vi "counter_control.vi"(0 "Signal-high duration":u32=20, 1 "Signal-high lead-up":u32=10) -> ()   [LabVIEW 2010]
panel:
  out "Configuration Error messages":T1
  # "Output"
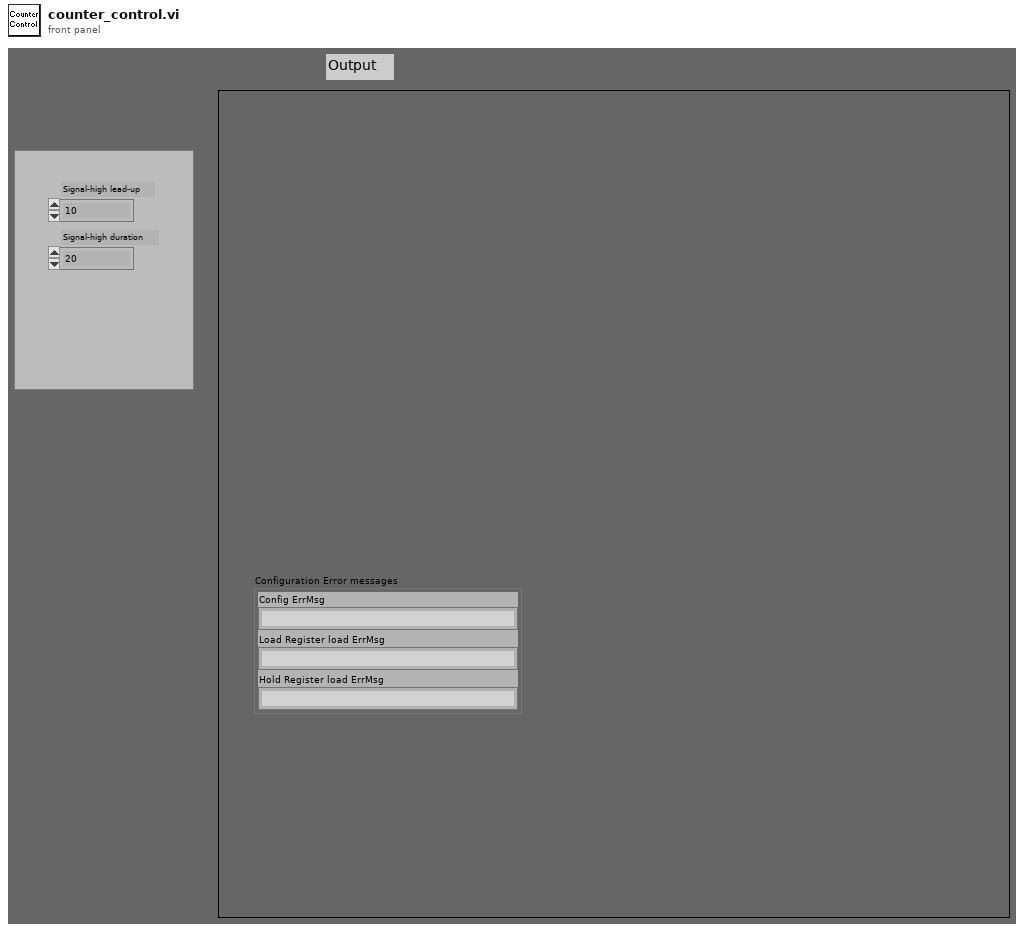
[diagram p1: front panel]
types:
  T1 = cluster{"Config ErrMsg":string, "Load Register load ErrMsg":string, "Hold Register load ErrMsg":string}
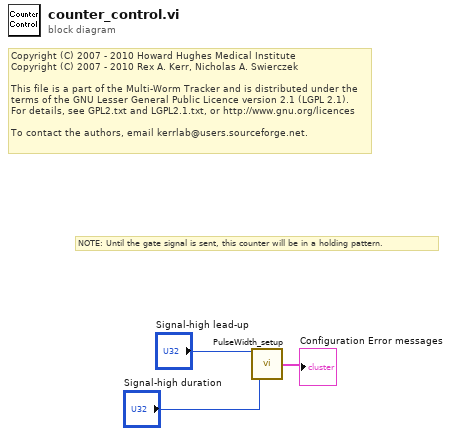
[diagram p0: block diagram]
diagram:
  # "Copyright (C) 2007 - 2010 Howard Hughes Medical Institute\nCopyright (C) 2007 - 2010 Rex A. Kerr, Nicholas A. Swierczek\n \nThis file is a part of the Multi-Worm Tracker and is distributed under the\nterms of the GNU Lesser General Public Licence version 2.1 (LGPL 2.1).\nFor details, see GPL2.txt and LGPL2.1.txt, or http://www.gnu.org/licences\n \nTo contact the authors, email kerrlab@users.sourceforge.net."
  # "NOTE: Until the gate signal is sent, this counter will be in a holding pattern."
  n1 = call "PulseWidth_setup.vi"("Signal-high duration"="Signal-high duration", "Signal-high lead-up"="Signal-high lead-up") -> ("Error output"=→"Configuration Error messages":T1)
